vi "MapPositionSend.vi"(8 "error in (no error)":errorcluster caption="错误输入（无错误）", 10 "MapPosition":T1, 11 "Voice in":refnum<class "Voice.lvclass">) -> (0 "error out":errorcluster caption="错误输出", 3 "Process State out":refnum<class "State Actor.lvclass">)   [LabVIEW 2014, in "States.lvlib" / "Voice.lvclass"]
uses:
  Voice.lvclass
  <vilib>/NI/Actors/State Actor/State Actor/State Actor.lvclass
  ctl/Point.ctl
  <vilib>/ActorFramework/Message Enqueuer/Message Enqueuer.lvclass/Message Enqueuer.ctl
  <vilib>/ActorFramework/Message Enqueuer/Enqueue.vi
  <vilib>/ActorFramework/Message Priority Queue/Priority Enqueue.vi
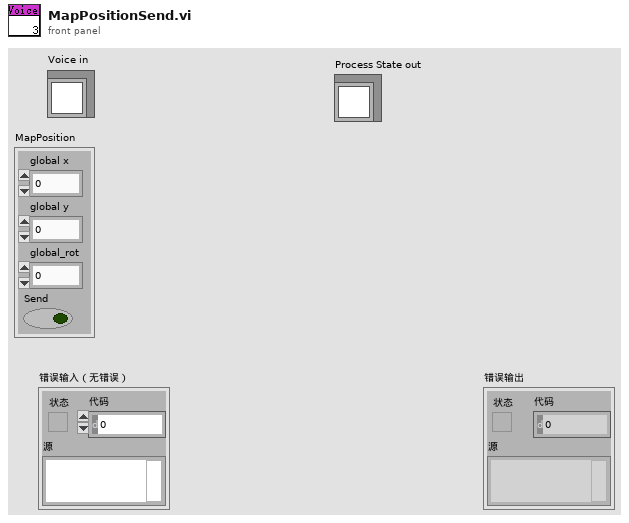
[diagram p1: front panel]
types:
  T1 = cluster{"global x":dbl, "global y":dbl, "global_rot":dbl, "Send":bool}
  T2 = typedef "Point.ctl" = cluster{"x":dbl, "y":dbl, "z":dbl}
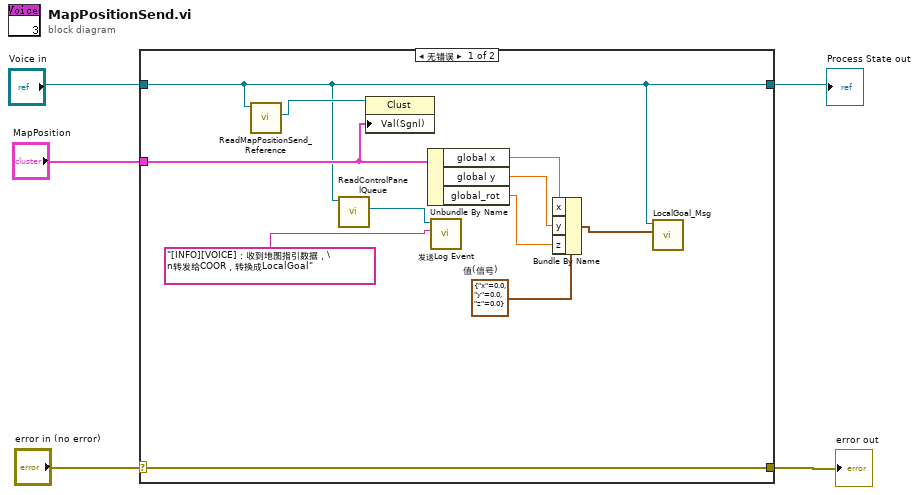
[diagram p0: block diagram]
diagram:
  n1 = case shown="无错误" "error in (no error)" {
    selector: "error in (no error)" -> [w16 w17]
    tunnel: [w16 w17] -> w4
    tunnel: [w6 w18] -> w2
    tunnel: "Voice in" -> [w6 w18]
    tunnel: "MapPosition" -> [w11 _]
    frame No Error {
      w12 = T2 {"x"=0.0, "y"=0.0, "z"=0.0}  # 值(信号)
      n2 = call-dynamic "ReadMapPositionSend_Reference.vi"("CoordinatorState输入"=w6) -> ("MapPositionSend_Reference"=w13:refnum<vi>)  [unwired: 8 in, 2 out]
      n3 = call-dynamic "ReadControlPanelQueue.vi"("CoordinatorState输入"=w6) -> ("操作者框架:消息待入队列"=w15:refnum<class "Message Enqueuer.lvclass">)  [unwired: 8 in, 2 out]
      n4 = property class="Clust"(reference=w13, "Val(Sgnl)"=w11) -> ()  [unwired: 1 in, 2 out]
      n5 = Unbundle By Name(w11) -> ("global x"=w10:dbl, "global y"=w9:dbl, "global_rot"=w8:dbl)
      n6 = call "发送Log Event.vi"("Event Text"="[INFO][VOICE]：收到地图指引数据，\n转发给COOR，转换成LocalGoal", "消息待入队列"=w15) -> ()  [unwired: 8 in, 2 out]
      n7 = Bundle By Name(cluster=w12, "x"=w10, "y"=w9, "z"=w8) -> (w7:T2)
      n8 = call-dynamic "LocalGoal_Msg.vi"("值(信号)"=w7, "Guiding 输入"=w6) -> ()  [unwired: 8 in, 2 out]
    }
    frame Error {
    }
  }
  "error out" <- w4
  "Process State out" <- w2
